vi "BarcodeprintR92A.vi"() -> ()   [LabVIEW 2020]
uses:
  Sources/Global_Variable/Global.vi
panel:
  out "error out":errorcluster
  in  "错误输入（无错误）":errorcluster
  in  "单选按钮":enum32{"保存", "打印"}(radio)=enum."打印"
  out "二维码图片":picture
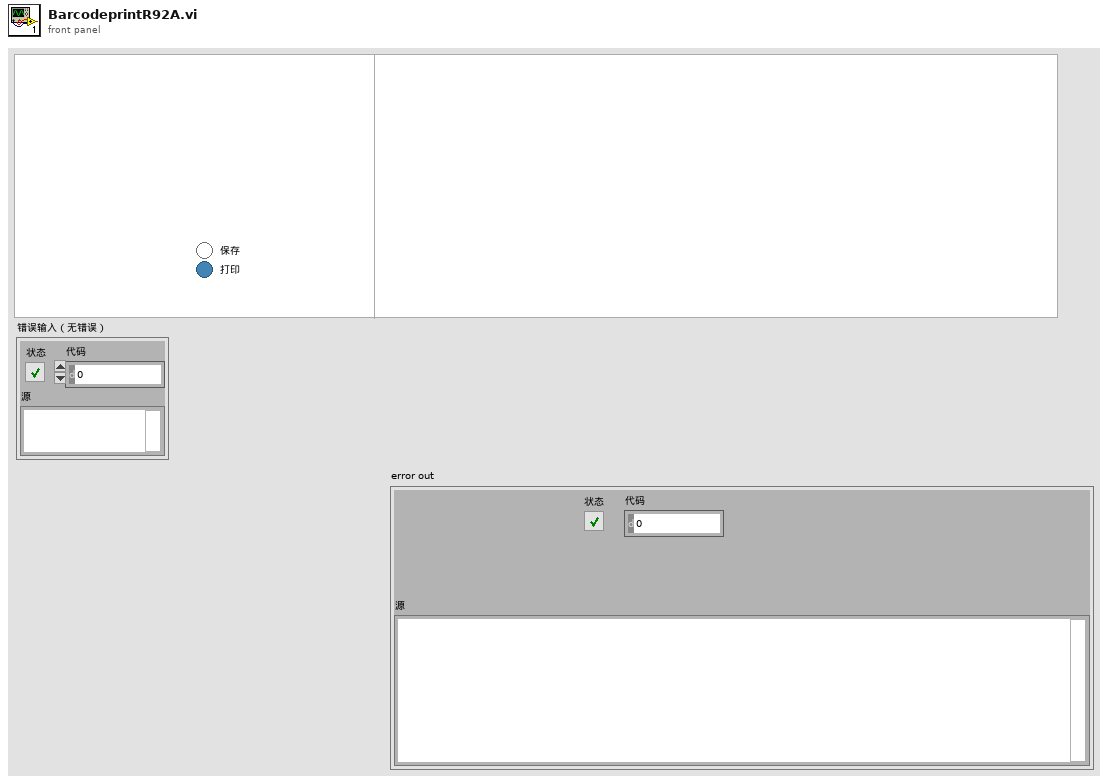
[diagram p1: front panel]
types:
  T1 = typedef "imagedata.ctl" = cluster{"image type":i32, "image depth":i32, "image":u8[], "mask":u8[], "colors":u32[], "Rectangle":cluster{"left":i16, "top":i16, "right":i16, "bottom":i16}}
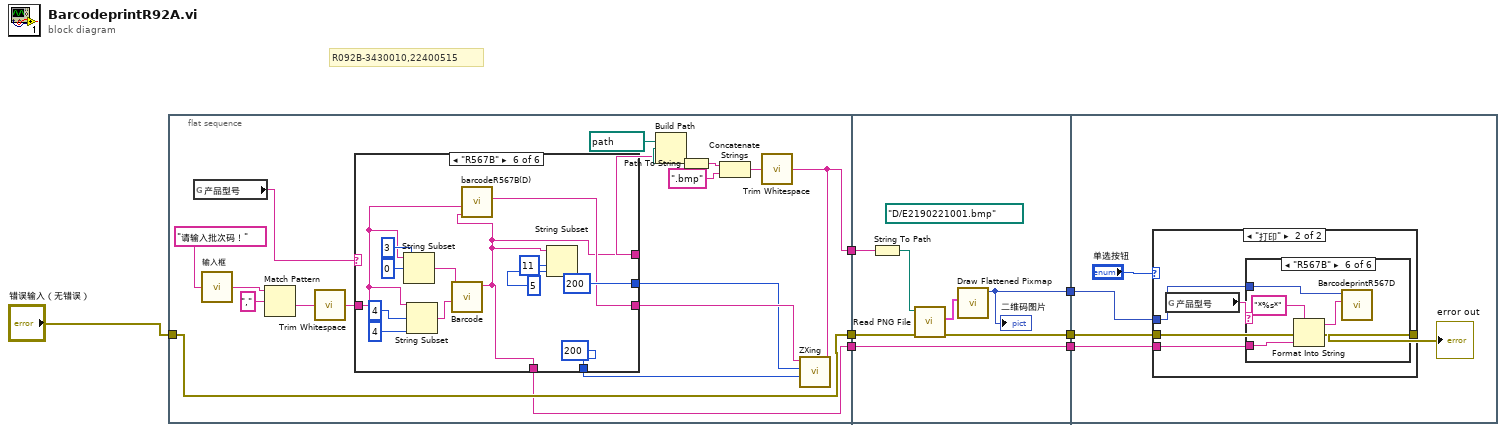
[diagram p0: block diagram]
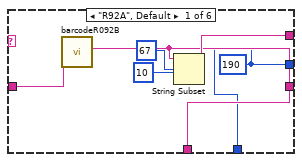
[diagram p2: hidden frame]
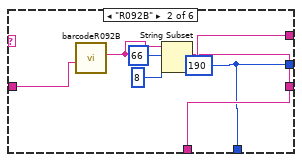
[diagram p3: hidden frame]
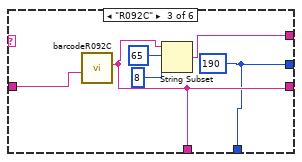
[diagram p4: hidden frame]
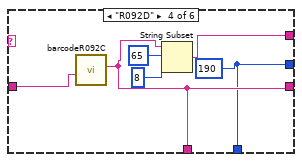
[diagram p5: hidden frame]
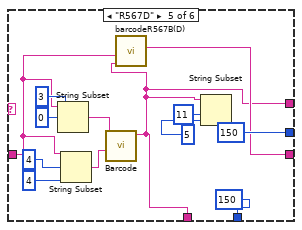
[diagram p6: hidden frame]
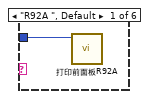
[diagram p8: hidden frame]
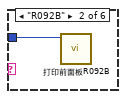
[diagram p9: hidden frame]
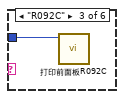
[diagram p10: hidden frame]
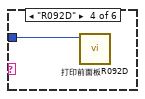
[diagram p11: hidden frame]
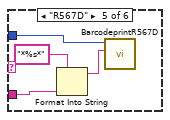
[diagram p12: hidden frame]
diagram:
  # "R092B-3430010,22400515"
  n1 = flat-sequence {
    tunnel: "错误输入（无错误）" -> [w25]
    tunnel: [w25] -> w5
    tunnel: [w11] -> w4
    tunnel: [w18] -> w1
    tunnel: w5 -> [w82]
    tunnel: [w80] -> w7
    tunnel: w4 -> [w79]
    tunnel: [w79] -> w3
    tunnel: [w78] -> w2
    tunnel: w1 -> [w77]
    tunnel: w7 -> [w86]
    tunnel: w3 -> [w84]
    tunnel: w2 -> [w83]
    frame #0 {
      n2 = global read "Global.vi" "产品型号"() -> (w14:string)
      n3 = call "输入框.vi"("提示信息"="请输入批次码！") -> ("条形码输出"=w15:string)
      n4 = Match Pattern(string=w15, regular expression="," ("正则表达式")) -> (after substring=w13:string)  [unwired: 1 in, 3 out]
      n5 = call <vilib>:"Trim Whitespace.vi"("string"=w13) -> ("trimmed string"=w10:string)  [unwired: 1 in]
      n6 = case shown="\"R567B\"" w14 {
        tunnel: [w31 w35 w41 w47 w50 w63] -> w19
        tunnel: w10 -> [w28 w34 w40 w46 w52 w65]
        tunnel: [w27 w33 w39 w45 w51 w64] -> w12
        tunnel: [w27 w33 w39 w45 w50 w63] -> w11
        tunnel: [w26 w32 w38 w44 150 ("width") 200 ("width")] -> w9
        tunnel: [w26 w32 w38 w44 150 ("height") 200 ("height")] -> w8
        frame "R92A", Default {
          w26 = 190 ("width")
          n7 = call "barcodeR092B.vi"("主码"=w28) -> ("R92A二维码"=w27:string)  [unwired: 9 in]
          n8 = String Subset(string=w27, offset (0)=67 ("偏移量(0)"), length (rest)=10 ("长度（剩余）")) -> (substring=w31:string)
        }
        frame "R092B" {
          w32 = 190 ("width")
          n9 = call "barcodeR092B.vi"("主码"=w34) -> ("R92A二维码"=w33:string)  [unwired: 9 in]
          n10 = String Subset(string=w33, offset (0)=66 ("偏移量(0)"), length (rest)=8 ("长度（剩余）")) -> (substring=w35:string)
        }
        frame "R092C" {
          w38 = 190 ("width")
          n11 = call "barcodeR092C.vi"("主码"=w40) -> ("R92A二维码"=w39:string)  [unwired: 9 in]
          n12 = String Subset(string=w39, offset (0)=65 ("偏移量(0)"), length (rest)=8 ("长度（剩余）")) -> (substring=w41:string)
        }
        frame "R092D" {
          w44 = 190 ("width")
          n13 = call "barcodeR092C.vi"("主码"=w46) -> ("R92A二维码"=w45:string)  [unwired: 9 in]
          n14 = String Subset(string=w45, offset (0)=65 ("偏移量(0)"), length (rest)=8 ("长度（剩余）")) -> (substring=w47:string)
        }
        frame "R567D" {
          n15 = String Subset(string=w52, offset (0)=0 ("偏移量(0)"), length (rest)=3 ("长度（剩余）")) -> (substring=w55:string)
          n16 = String Subset(string=w52, offset (0)=4 ("偏移量(0)"), length (rest)=4 ("长度（剩余）")) -> (substring=w56:string)
          n17 = call "Barcode.vi"("流水号"=w56, "年月日"=w55) -> ("条形码"=w50:string)  [unwired: 9 in]
          n18 = call "barcodeR567B(D).vi"("规则码"=w50, "主码"=w52) -> ("R567D(B)二维码"=w51:string)  [unwired: 7 in, 1 out]
          n19 = String Subset(string=w50, offset (0)=11 ("偏移量(0)"), length (rest)=5 ("长度（剩余）")) -> ()  [unwired: 1 out]
        }
        frame "R567B" {
          n20 = String Subset(string=w65, offset (0)=0 ("偏移量(0)"), length (rest)=3 ("长度（剩余）")) -> (substring=w68:string)
          n21 = String Subset(string=w65, offset (0)=4 ("偏移量(0)"), length (rest)=4 ("长度（剩余）")) -> (substring=w69:string)
          n22 = call "Barcode.vi"("流水号"=w69, "年月日"=w68) -> ("条形码"=w63:string)  [unwired: 9 in]
          n23 = call "barcodeR567B(D).vi"("规则码"=w63, "主码"=w65) -> ("R567D(B)二维码"=w64:string)  [unwired: 7 in, 1 out]
          n24 = String Subset(string=w63, offset (0)=11 ("偏移量(0)"), length (rest)=5 ("长度（剩余）")) -> ()  [unwired: 1 out]
        }
      }
      n25 = Build Path(base path=path "D:/条码" ("基路径"), name or relative path=w19) -> (appended path=w22:path)
      n26 = Path To String(path=w22) -> (string=w20:string)
      n27 = Concatenate Strings(w20, ".bmp" ("字符串")) -> (w21:string)
      n28 = call <vilib>:"Trim Whitespace.vi"("string"=w21) -> ("trimmed string"=w18:string)  [unwired: 1 in]
      n29 = call "ZXing.vi"("二维码保存路径"=w18, "height"=w8, "width"=w9, "contents"=w12) -> ()  [unwired: 7 in, 1 out]
    }
    frame #1 {
      (unwired) path "D:/E2190221001.bmp" ("path to BMP file")
      n30 = String To Path(string=w77) -> (path=w76:path)
      n31 = call <vilib>:"Read PNG File.vi"("error in (no error)"=w82, "path to PNG file"=w76) -> ("error out"=w80:errorcluster, "image data"=w81:T1)  [unwired: 7 in, 1 out]
      n32 = call <vilib>:"Draw Flattened Pixmap.vi"("image data"=w81) -> ("new picture"=w78:picture)  [unwired: 8 in]
      "二维码图片" <- w78
    }
    frame #2 {
      n33 = case shown="\"打印\"" "单选按钮" {
        tunnel: w86 -> [w88 w92]
        tunnel: [w88 w92] -> w85
        tunnel: w84 -> [_ w90]
        tunnel: w83 -> [_ w91]
        frame "保存", Default {
        }
        frame "打印" {
          n34 = global read "Global.vi" "产品型号"() -> (w89:string)
          n35 = case shown="\"R567B\"" w89 {
            tunnel: w91 -> [w93 w94 w95 w96 w100 w104]
            tunnel: w90 -> [_ _ _ _ w98 w102]
            frame "R92A ", Default {
              n36 = call "打印前面板R92A.vi"("二维图片"=w93) -> ()  [unwired: 10 in]
            }
            frame "R092B" {
              n37 = call "打印前面板R092B.vi"("二维图片"=w94) -> ()  [unwired: 10 in]
            }
            frame "R092C" {
              n38 = call "打印前面板R092C.vi"("二维图片"=w95) -> ()  [unwired: 10 in]
            }
            frame "R092D" {
              n39 = call "打印前面板R092D.vi"("二维图片"=w96) -> ()  [unwired: 10 in]
            }
            frame "R567D" {
              n40 = Format Into String(format string="*%s*" ("格式字符串"), w98) -> (resulting string=w97:string)  [unwired: 2 in, 1 out]
              n41 = call "BarcodeprintR567D.vi"("二维图片 2"=w100, "字符串"=w97) -> ()  [unwired: 9 in]
            }
            frame "R567B" {
              n42 = Format Into String(format string="*%s*" ("格式字符串"), w102) -> (resulting string=w101:string)  [unwired: 2 in, 1 out]
              n43 = call "BarcodeprintR567D.vi"("二维图片 2"=w104, "字符串"=w101) -> ()  [unwired: 9 in]
            }
          }
        }
      }
      "error out" <- w85
    }
  }
